vi "Array.vi"() -> ()   [LabVIEW 2017]
panel:
  out "添加的数组":i32[](array[numeric])
  out "子数组":i32[](array[numeric])
  out "大小":i32[](array[numeric])
  out "数组 6":i32[][](array[numeric])
  out "数组 5":i32[][](array[numeric])
  out "数组 4":i32[](array[numeric])
  out "数值":i32
  out "数组 3":i32[](array[numeric])
  in  "数组 2":string[][](array[string])
  in  "数组":dbl[](array[numeric])
  # "循环中有两种结构通道：索引和最终值"
  # "二维数组"
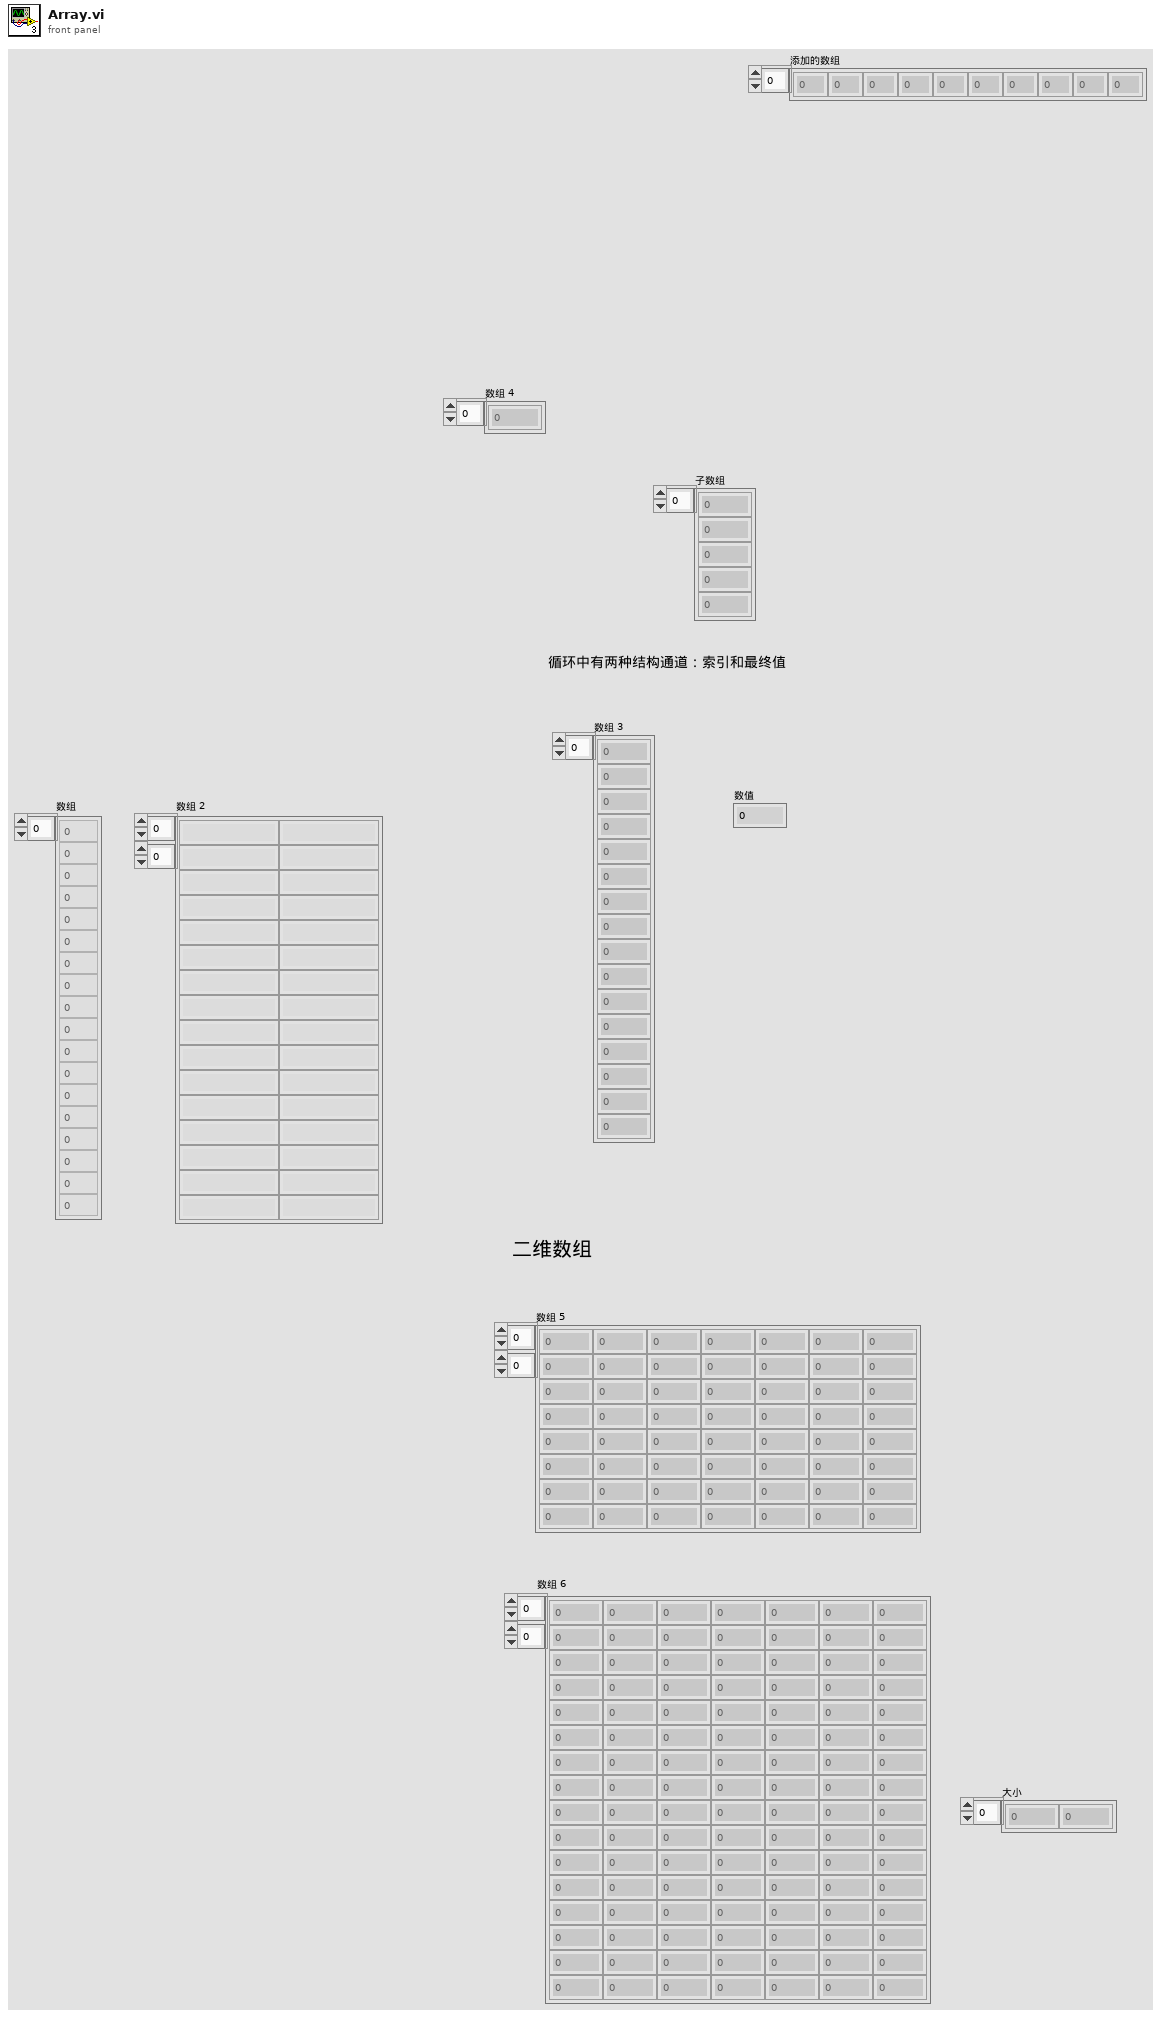
[diagram p1: front panel]
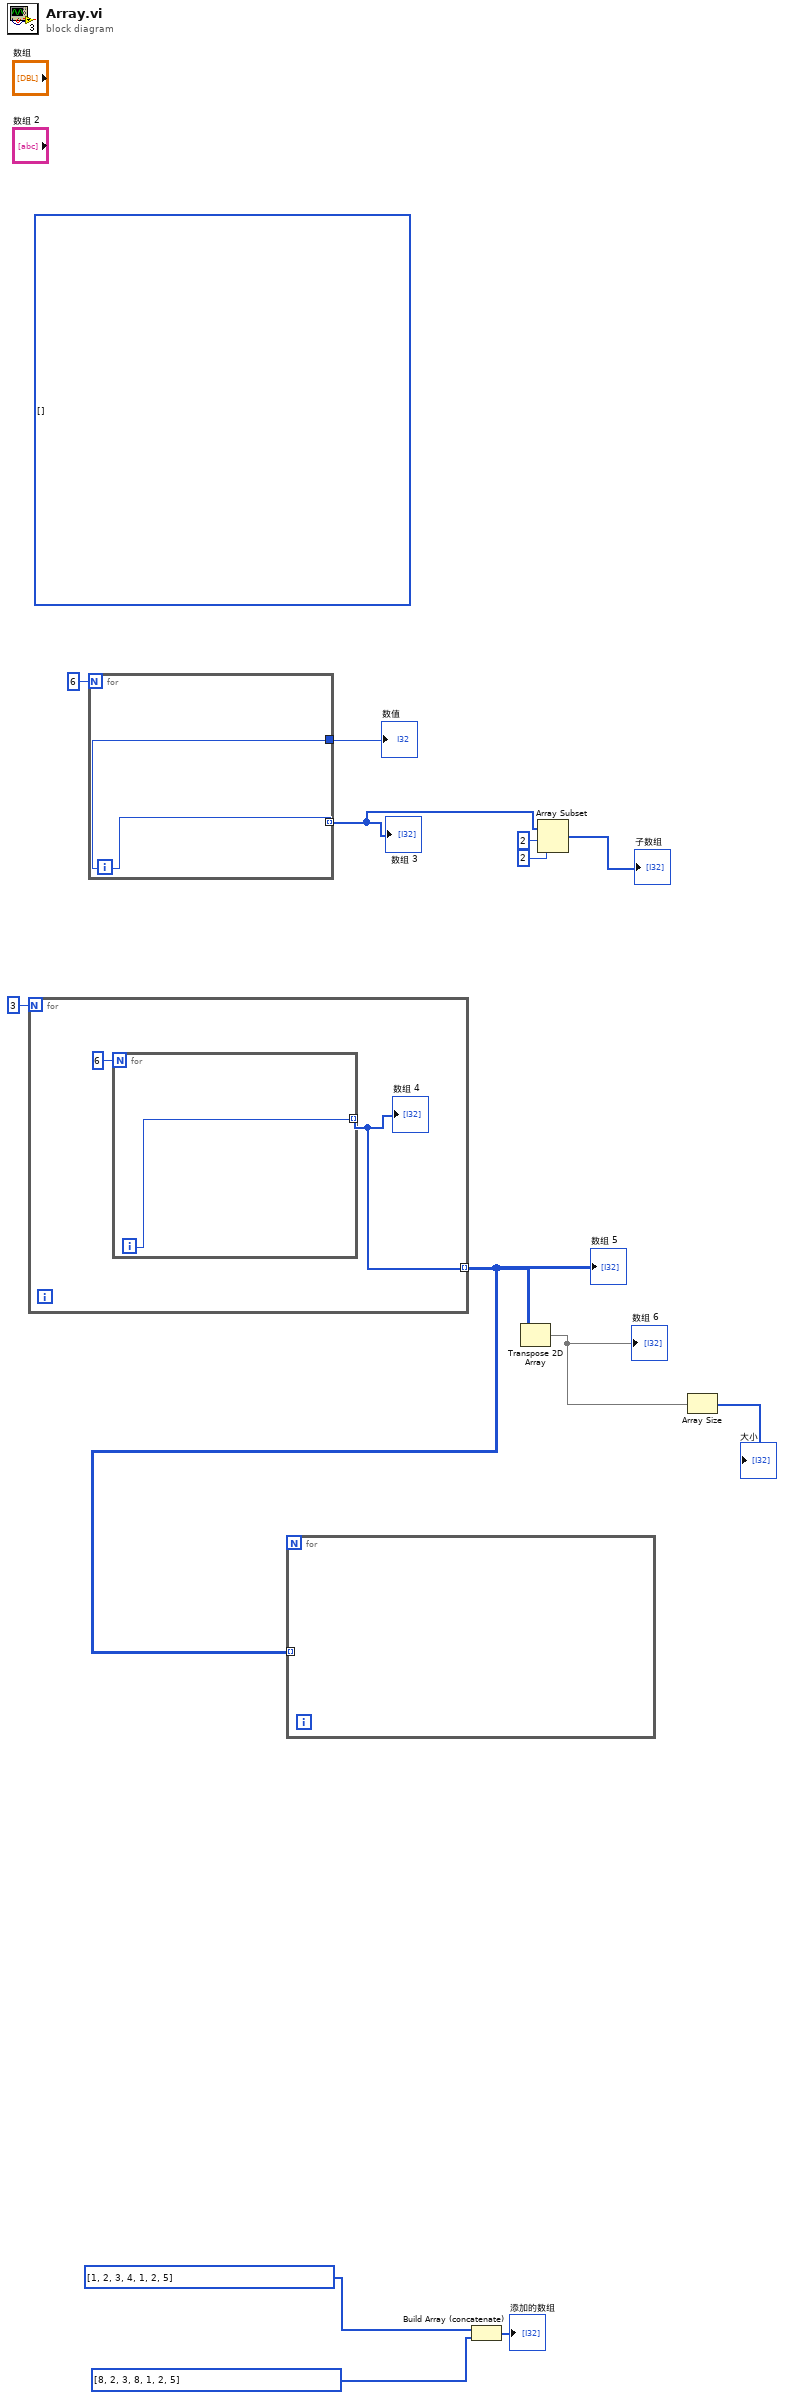
[diagram p0: block diagram]
diagram:
  (unwired) i32[][][] []
  n1 = for {
    N: 3 -> [_]
    tunnel: [w14] -> w8 mode=indexing
    n2 = for {
      N: 6 -> [_]
      tunnel: [w16] -> w14 mode=indexing
      i -> [w16]
    }
    "数组 4" <- w14
  }
  "数组 5" <- w8
  n3 = for {
    N: 6 -> [_]
    tunnel: [w17] -> w12
    tunnel: [w17] -> w7 mode=indexing
    i -> [w17]
  }
  "数组 3" <- w7
  "数值" <- w12
  n4 = for {
    tunnel: w8 -> [_] mode=indexing
  }
  n5 = Build Array (concatenate)(i32[] [1, 2, 3, 4, 1, 2, 5], i32[] [8, 2, 3, 8, 1, 2, 5]) -> (→"添加的数组":i32[])
  n6 = Transpose 2D Array(2D array=w8) -> (transposed array=w10:i32[][])
  "数组 6" <- w10
  n7 = Array Subset(array=w7, index=2 ("索引"), length=2 ("长度")) -> (→"子数组":i32[])
  n8 = Array Size(array=w10) -> (size(s)=→"大小":i32[])
